vi "Configure Offset Angle.vi"(8 "error in (no error)":errorcluster, 10 "ccw offset angle (rad)":dbl, 11 "NI_Robotics_Starter Kit Servo Motor in":refnum<class "NI_Robotics_Starter Kit Servo Motor.lvclass">) -> (0 "error out":errorcluster, 3 "NI_Robotics_Starter Kit Servo Motor out":refnum<class "NI_Robotics_Starter Kit Servo Motor.lvclass">)   [LabVIEW 2017, in "NI_Robotics_Starter Kit Servo Motor.lvclass"]
uses:
  <vilib>/robotics/Starter Kit/Servo Motor/NI_Robotics_Starter Kit Servo Motor.lvclass
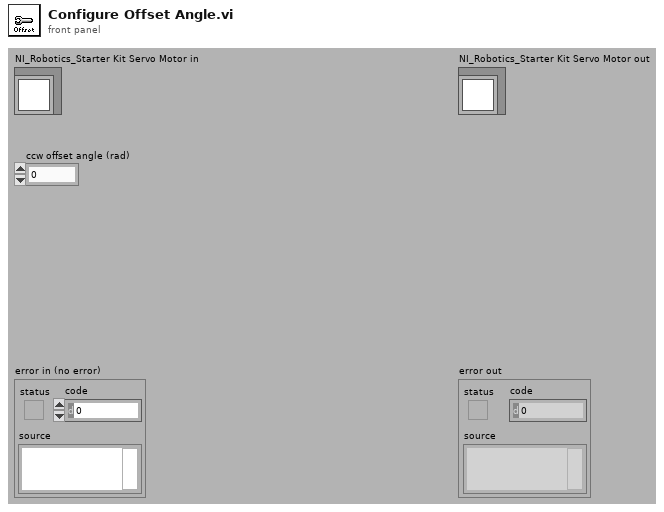
[diagram p1: front panel]
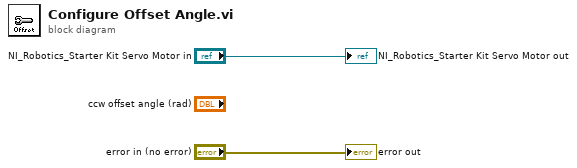
[diagram p0: block diagram]
diagram:
  "error out" <- "error in (no error)"
  "NI_Robotics_Starter Kit Servo Motor out" <- "NI_Robotics_Starter Kit Servo Motor in"
